vi "Periodic Tasks.vi"(8 "error in":errorcluster) -> ()   [LabVIEW 2014]
doc: "This VI runs in parallel to other tasks. It can contain as many user-defined periodic loops as you need. These can carry out PID or other sorts of timed response."
uses:
  <vilib>/Rock Robotics/WPI/Solenoid/WPI_SolenoidValue.ctl
  <vilib>/Rock Robotics/WPI/Joystick/WPI_JoystickGetSetRefNum.vi
  <vilib>/Rock Robotics/WPI/RobotDrive/WPI_RobotDriveGetSetRefNum.vi
  Global 1.vi
  <vilib>/Rock Robotics/WPI/Solenoid/WPI_SolenoidSetEnum.vi
  <vilib>/Rock Robotics/Network Tables/SD Write Numeric Array.vi
  <vilib>/Rock Robotics/Network Tables/SD Write Number.vi
  <vilib>/Rock Robotics/Network Tables/SD Read Boolean.vi
  <vilib>/addons/control/pid/pid.llb/PID (DBL).vi
  <vilib>/addons/control/pid/NI_PID_pid.lvlib
panel:
  out "Switch Pressed":bool
  out "Fudge":dbl
  out "Potentiometer Voltage":dbl
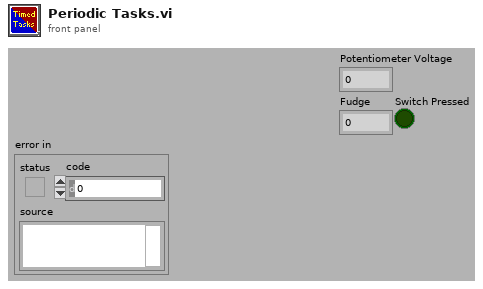
[diagram p1: front panel]
types:
  T1 = typedef "WPI_EncoderDevRef.ctl" = cluster{"DevStatus":errorcluster, "EncoderIndex":T2, "CounterIndex":T3, "DistancePerCount":dbl, "Decoding Type":T4}
  T2 = typedef "FPGA_EncoderIdx.ctl" = enum8{"Enc 0", "Enc 1", "Enc 2", "Enc 3", "Enc 4", "Enc 5", "Enc 6", "Enc 7", "Invalid"}
  T3 = typedef "FPGA_CounterCtrSystemIndex.ctl" = enum8{"Ctr 0", "Ctr 1", "Ctr 2", "Ctr 3", "Ctr 4", "Ctr 5", "Ctr 6", "Ctr 7", "Invalid"}
  T4 = typedef "WPI_EncoderType.ctl" = enum16{"1x", "2x", "4x"}
  T5 = typedef "WPI_JoystickDevRef.ctl" = cluster{"Device":T6}
  T6 = typedef "WPI_JoystickDeviceEnum.ctl" = enum16{"USB 0", "USB 1", "USB 2", "USB 3", "USB 4", "USB 5"}
  T7 = typedef "WPI_RobotDriveDevRef.ctl" = cluster{"DevStatus":errorcluster, "Motors[]":T8[], "Square Inputs":bool, "Max Output":dbl}
  T8 = typedef "WPI_MotorControlDeviceRef.ctl" = cluster{"DeviceStatus":errorcluster, "Type":T9, "PWM":cluster{"Controller":T10, "PWM Channel":T11, "DeadBand":T12}, "CAN":cluster{"Device Number":u8, "Control Mode":T13, "Semaphore":T14, "Max Vout":dbl, "TalonSRX Control Mode":T15}, "Invert":bool, "TransformRef":T16, "InvTransformRef":T16}
  T9 = typedef "WPI_MotorControlType.ctl" = enum16{"PWM", "CAN", "CANTalonSRX"}
  T10 = typedef "FPGA_TypedefDigitalModule.ctl" = enum16{"Controller 1"}
  T11 = typedef "FPGA_DIOPWMChannel.ctl" = enum8{"PWM 0", "PWM 1", "PWM 2", "PWM 3", "PWM 4", "PWM 5", "PWM 6", "PWM 7", "PWM 8", "PWM 9", "PWM MXP 0", "PWM MXP 1", "PWM MXP 2", "PWM MXP 3", "PWM MXP 4", "PWM MXP 5", "PWM MXP 6", "PWM MXP 7", "PWM MXP 8", "PWM MXP 9", "Invalid"}
  T12 = typedef "WPI_PWMDeadband.ctl" = cluster{"Name":string, "maxPositivePwm":i32, "minPositivePwm":i32, "centerPwm":i32, "maxNegativePwm":i32, "minNegativePwm":i32, "angularRange":u16}
  T13 = typedef "WPI_CANJaguar_ControlMode.ctl" = enum8{"Percent VBus", "Current", "Speed", "Position", "Voltage"}
  T14 = typedef "Semaphore RefNum" = refnum<k1>
  T15 = typedef "WPI_CANTalonSRX_APIControlMode.ctl" = enum8{"Percent VBus", "Speed", "Position", "Slave", "Unchanged / Invalid"}
  T16 = typedef "WPI_PWMTransform_ConPane.ctl" = refnum<vi>
  T17 = cluster{"JoystickDevRef":T5, "RobotDriveDevRef":T7}
  T18 = cluster{"proportional gain (Kc)":dbl, "integral time (Ti, min)":dbl, "derivative time (Td, min)":dbl}
  T19 = typedef "WPI_SolenoidValue.ctl" = enum16{"Off", "On", "Forward", "Reverse"}
  T20 = typedef "WPI_SolenoidDevRef.ctl" = cluster{"DevStatus":errorcluster, "Pneumatics Control Module":u8, "Forward Solenoid Channel":T21, "Reverse Solenoid Channel":T21}
  T21 = typedef "WPI_SolenoidChannel.ctl" = enum8{"Solenoid 0", "Solenoid 1", "Solenoid 2", "Solenoid 3", "Solenoid 4", "Solenoid 5", "Solenoid 6", "Solenoid 7", "Invalid"}
  T22 = typedef "WPI_SwitchDevRef.ctl" = cluster{"DevStatus":errorcluster, "DIO Channel":T23, "Controller":T10, "CntIndex":T3, "Normally Closed":bool}
  T23 = typedef "FPGA_DIOChannel.ctl" = enum8{"DIO 0", "DIO 1", "DIO 2", "DIO 3", "DIO 4", "DIO 5", "DIO 6", "DIO 7", "DIO 8", "DIO 9", "DIO MXP 0", "DIO MXP 1", "DIO MXP 2", "DIO MXP 3", "DIO MXP 4", "DIO MXP 5", "DIO MXP 6", "DIO MXP 7", "DIO MXP 8", "DIO MXP 9", "DIO MXP 10", "DIO MXP 11", "DIO MXP 12", "DIO MXP 13", "DIO MXP 14", "DIO MXP 15", "Invalid"}
  T24 = typedef "WPI_PotentiometerDevRef.ctl" = cluster{"DevStatus":errorcluster, "Controller":T25, "Analog Channel":T26, "Invert Output":bool}
  T25 = typedef "FPGA_TypedefAnalogModule.ctl" = enum16{"Controller 1"}
  T26 = typedef "FPGA_AIChannel.ctl" = enum8{"AI 0", "AI 1", "AI 2", "AI 3", "AI MXP 0", "AI MXP 1", "AI MXP 2", "AI MXP 3", "Invalid"}
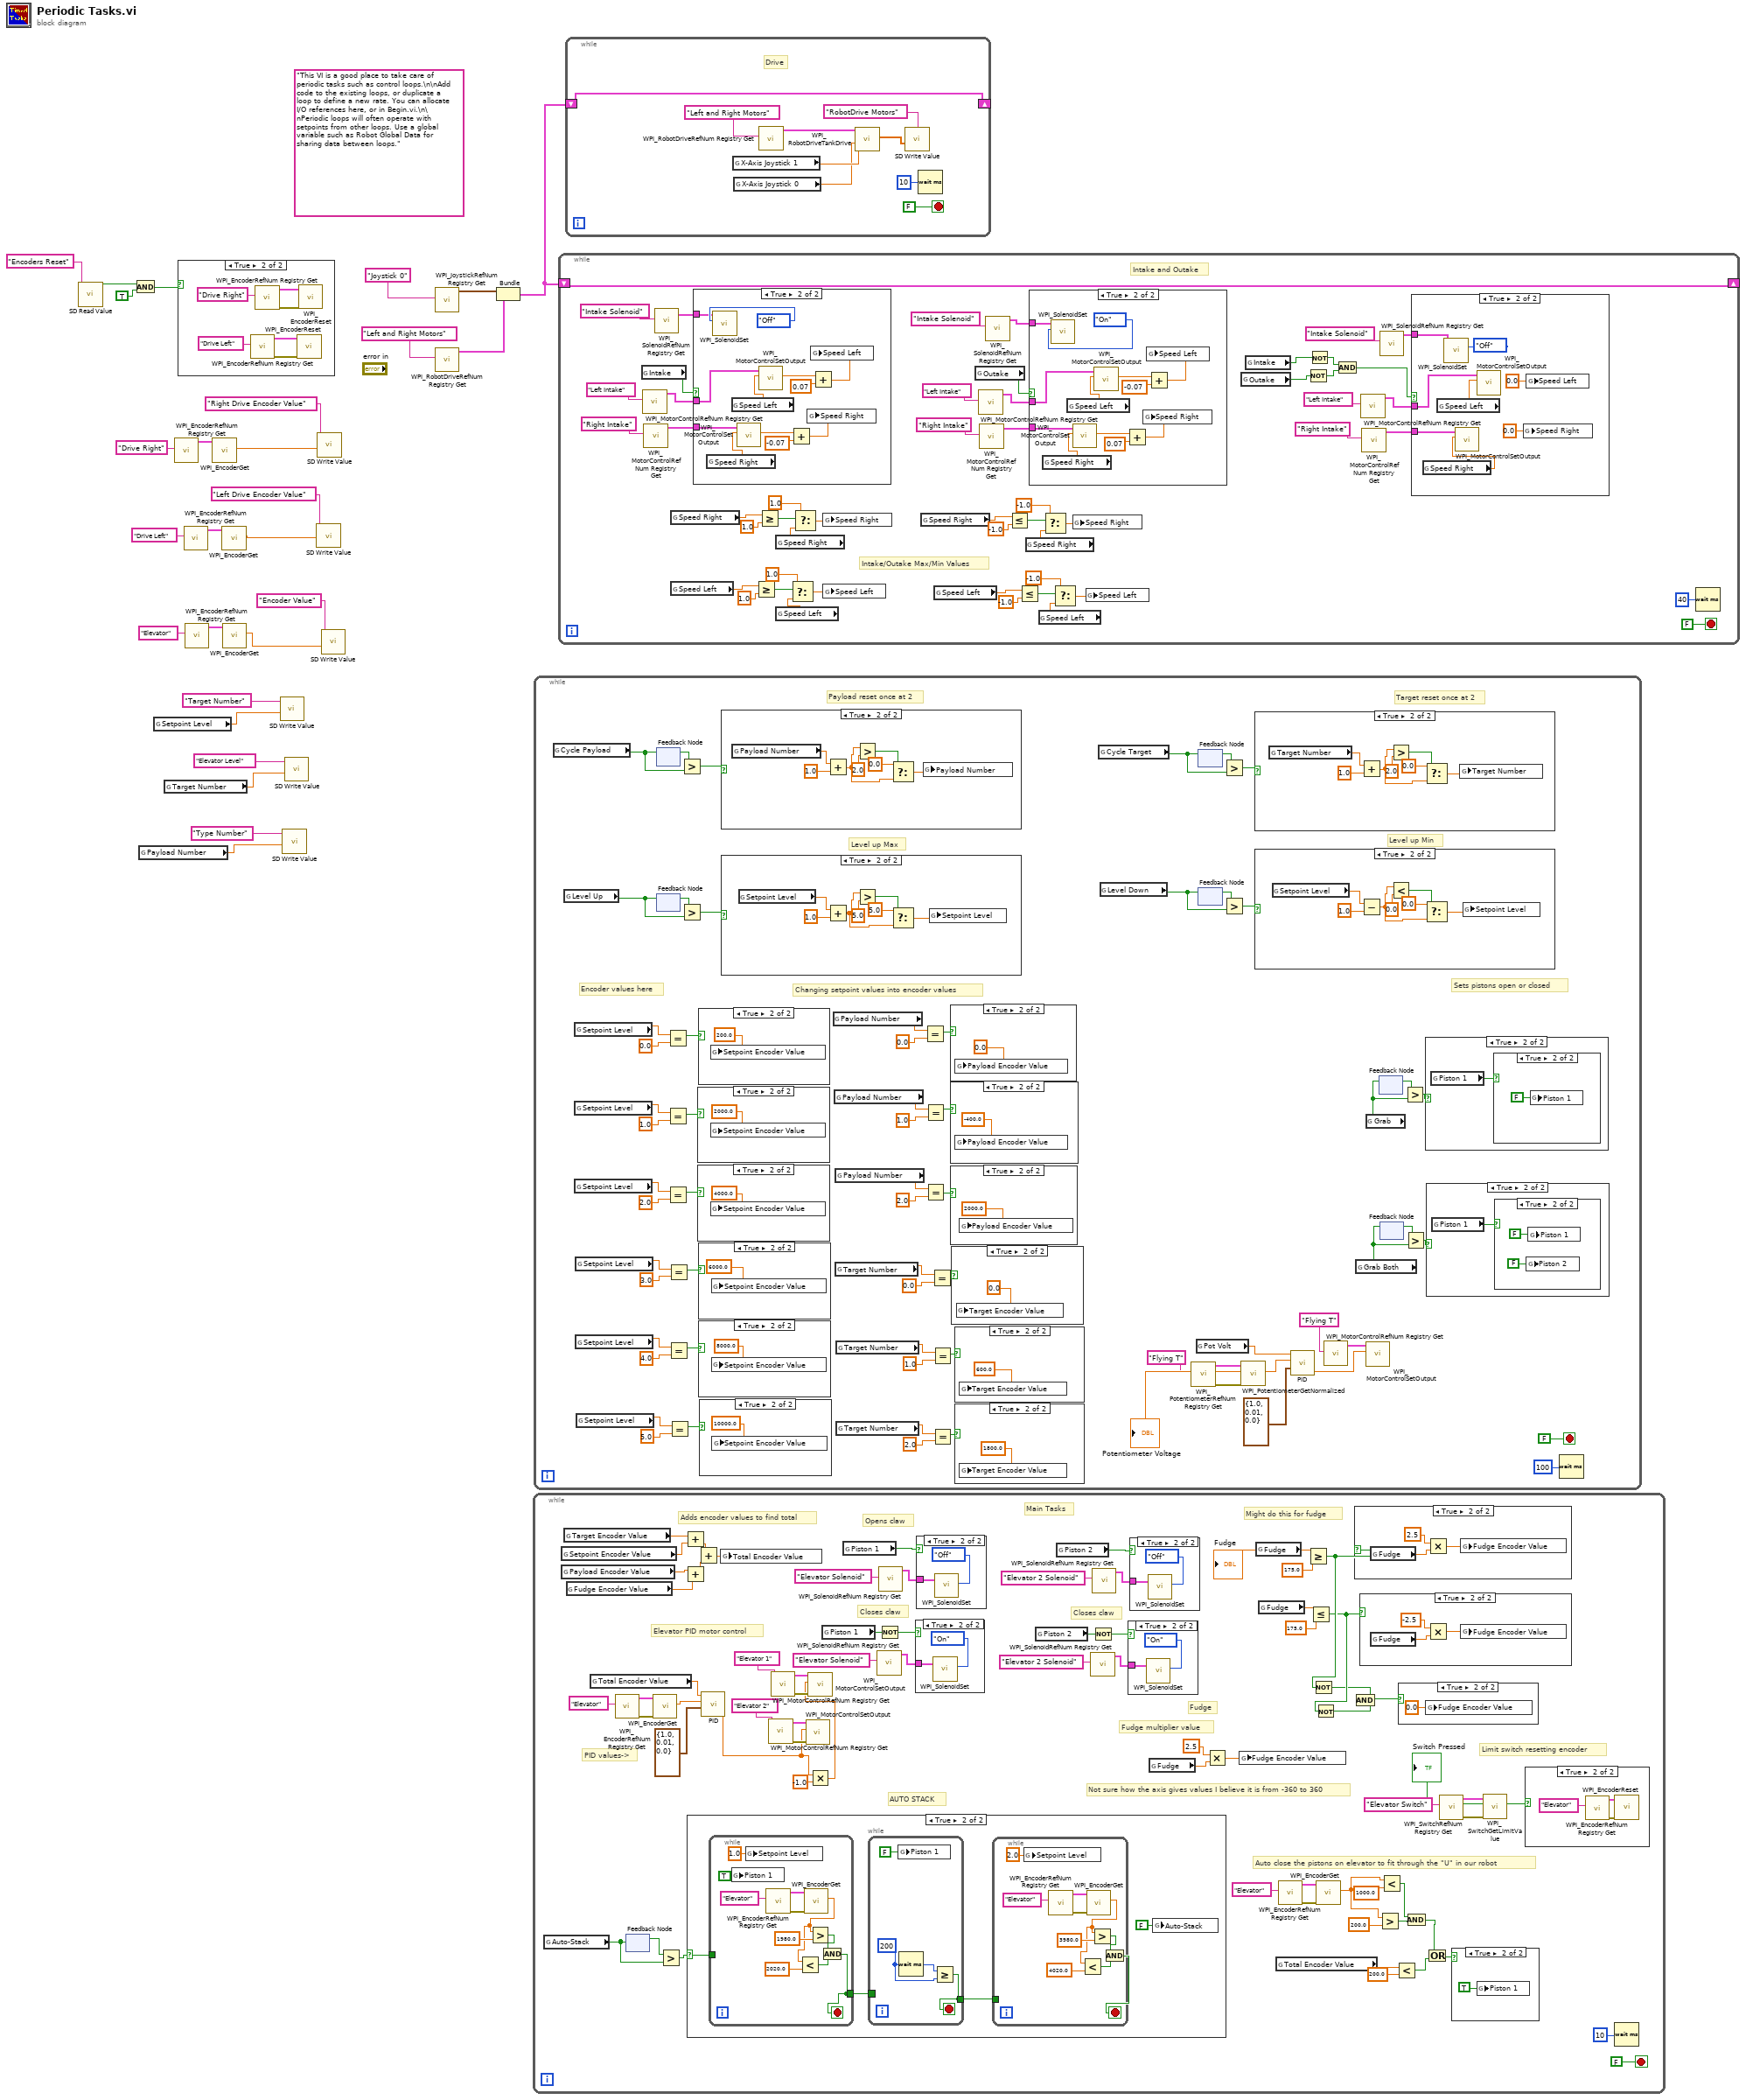
[diagram p0: block diagram]
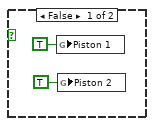
[diagram p14: hidden frame]
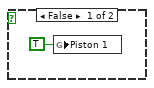
[diagram p16: hidden frame]
diagram:
  (unwired) "This VI is a good place to take care of periodic tasks such as control loops.\n\nAdd code to the existing loops, or duplicate a loop to define a new rate. You can allocate I/O references here, or in Begin.vi.\n\nPeriodic loops will often operate with setpoints from other loops. Use a global variable such as Robot Global Data for sharing data between loops."
  n1 = call-poly <vilib>:"SD Read Value.vi"("Name"="Encoders Reset") -> ("Boolean"=w2:bool)  [unwired: 8 in, 2 out]
  n2 = And(x=w2, y=TRUE) -> (x .and. y?=w1:bool)
  n3 = global read "Global 1.vi" "Payload Number"() -> (w7:dbl)
  n4 = global read "Global 1.vi" "Setpoint Level"() -> (w5:dbl)
  n5 = global read "Global 1.vi" "Target Number"() -> (w6:dbl)
  n6 = call <vilib>:"WPI_EncoderRefNum Registry Get.vi"("refnum name"="Drive Right") -> ("EncoderDevRef"=w19:T1)  [unwired: 9 in, 1 out]
  n7 = case shown="True" w1 {
    frame False {
    }
    frame True {
      n8 = call <vilib>:"WPI_EncoderRefNum Registry Get.vi"("refnum name"="Drive Left") -> ("error out"=w28:errorcluster, "EncoderDevRef"=w29:T1)  [unwired: 9 in]
      n9 = call <vilib>:"WPI_EncoderRefNum Registry Get.vi"("refnum name"="Drive Right") -> ("error out"=w31:errorcluster, "EncoderDevRef"=w30:T1)  [unwired: 9 in]
      n10 = call <vilib>:"WPI_EncoderReset.vi"("error in (no error)"=w28, "EncoderDevRef"=w29) -> ()  [unwired: 8 in, 2 out]
      n11 = call <vilib>:"WPI_EncoderReset.vi"("error in (no error)"=w31, "EncoderDevRef"=w30) -> ()  [unwired: 8 in, 2 out]
    }
  }
  n12 = call <vilib>:"WPI_EncoderRefNum Registry Get.vi"("refnum name"="Drive Left") -> ("EncoderDevRef"=w16:T1)  [unwired: 9 in, 1 out]
  n13 = call <vilib>:"WPI_EncoderRefNum Registry Get.vi"("refnum name"="Elevator") -> ("EncoderDevRef"=w14:T1)  [unwired: 9 in, 1 out]
  n14 = call <vilib>:"WPI_EncoderGet.vi"("EncoderDevRef"=w19) -> ("Distance"=w17:dbl)  [unwired: 5 in, 5 out]
  n15 = call <vilib>:"WPI_EncoderGet.vi"("EncoderDevRef"=w16) -> ("Distance"=w11:dbl)  [unwired: 5 in, 5 out]
  n16 = call <vilib>:"WPI_EncoderGet.vi"("EncoderDevRef"=w14) -> ("Distance"=w12:dbl)  [unwired: 5 in, 5 out]
  n17 = call-poly <vilib>:"SD Write Value.vi"("Numeric"=w5, "Name"="Target Number") -> ()  [unwired: 8 in, 2 out]
  n18 = call-poly <vilib>:"SD Write Value.vi"("Numeric"=w7, "Name"="Type Number") -> ()  [unwired: 8 in, 2 out]
  n19 = call-poly <vilib>:"SD Write Value.vi"("Numeric"=w6, "Name"="Elevator Level") -> ()  [unwired: 8 in, 2 out]
  n20 = call-poly <vilib>:"SD Write Value.vi"("Numeric"=w11, "Name"="Left Drive Encoder Value") -> ()  [unwired: 8 in, 2 out]
  n21 = call-poly <vilib>:"SD Write Value.vi"("Numeric"=w17, "Name"="Right Drive Encoder Value") -> ()  [unwired: 8 in, 2 out]
  n22 = call-poly <vilib>:"SD Write Value.vi"("Numeric"=w12, "Name"="Encoder Value") -> ()  [unwired: 8 in, 2 out]
  n23 = call <vilib>:"WPI_JoystickRefNum Registry Get.vi"("refnum name"="Joystick 0") -> ("JoystickDevRef"=w25:T5)  [unwired: 1 in, 9 out]
  n24 = call <vilib>:"WPI_RobotDriveRefNum Registry Get.vi"("refnum name"="Left and Right Motors") -> ("RobotDriveDevRef"=w24:T7)  [unwired: 1 in, 9 out]
  n25 = Bundle("JoystickDevRef"=w25, "RobotDriveDevRef"=w24) -> (w23:T17)  [unwired: 1 out]
  n26 = while {
    stop <- FALSE stop-if-true
    # "Auto close the pistons on elevator to fit through the \"U\" in our robot"
    # "Closes claw"
    # "Main Tasks"
    # "Limit switch resetting encoder"
    # "AUTO STACK"
    # "Might do this for fudge"
    # "Not sure how the axis gives values I believe it is from -360 to 360"
    # "Fudge multiplier value"
    # "Fudge"
    # "Elevator PID motor control"
    # "Adds encoder values to find total"
    # "Closes claw"
    # "Opens claw"
    # "PID values->"
    n27 = global read "Global 1.vi" "Auto-Stack"() -> (w61:bool)
    n28 = global read "Global 1.vi" "Setpoint Encoder Value"() -> (w100:dbl)
    n29 = global read "Global 1.vi" "Payload Encoder Value"() -> (w79:dbl)
    n30 = global read "Global 1.vi" "Target Encoder Value"() -> (w101:dbl)
    n31 = global read "Global 1.vi" "Fudge Encoder Value"() -> (w78:dbl)
    n32 = global read "Global 1.vi" "Total Encoder Value"() -> (w88:dbl)
    n33 = call <vilib>:"WPI_EncoderRefNum Registry Get.vi"("refnum name"="Elevator") -> ("error out"=w93:errorcluster, "EncoderDevRef"=w92:T1)  [unwired: 9 in]
    n34 = feedback-in #1(w61) -> ()
    n35 = feedback #1() -> (w62:bool)  [unwired: 1 in]
    n36 = call <vilib>:"WPI_EncoderGet.vi"("error in (no error)"=w93, "EncoderDevRef"=w92) -> ("Distance"=w89:dbl)  [unwired: 4 in, 5 out]
    n37 = Greater?(x=w62, y=w61) -> (0:w60:bool)
    n38 = Add(x=w101, y=w100) -> (x+y=w76:dbl)
    n39 = Add(x=w79, y=w78) -> (x+y=w77:dbl)
    n40 = case shown="True" w60 {
      selector: w60 -> [_ w115]
      frame False {
      }
      frame True {
        n41 = while {
          tunnel: w115 -> [_]
          tunnel: [w130] -> w114
          stop <- w130 stop-if-true
          n42 = global write "Global 1.vi" "Piston 1"(TRUE) -> ()
          n43 = global write "Global 1.vi" "Setpoint Level"(1.0 ("Setpoint Level")) -> ()
          n44 = call <vilib>:"WPI_EncoderRefNum Registry Get.vi"("refnum name"="Elevator") -> ("error out"=w138:errorcluster, "EncoderDevRef"=w137:T1)  [unwired: 9 in]
          n45 = call <vilib>:"WPI_EncoderGet.vi"("error in (no error)"=w138, "EncoderDevRef"=w137) -> ("Distance"=w134:dbl)  [unwired: 4 in, 5 out]
          n46 = Less?(x=w134, y=2020.0) -> (x < y?=w131:bool)
          n47 = Greater?(x=w134, y=1980.0) -> (0:w132:bool)
          n48 = And(x=w132, y=w131) -> (x .and. y?=w130:bool)
        }
        n49 = while {
          tunnel: w114 -> [_]
          tunnel: [w126] -> w113
          stop <- w126 stop-if-true
          w127 = u32 200 ("milliseconds to wait")
          n50 = global write "Global 1.vi" "Piston 1"(FALSE) -> ()
          n51 = Wait (ms)(milliseconds to wait=w127) -> (millisecond timer value=w128:u32)
          n52 = Greater Or Equal?(x=w128, y=w127) -> (x >= y?=w126:bool)
        }
        n53 = while {
          tunnel: w113 -> [_]
          stop <- w116 stop-if-true
          n54 = global write "Global 1.vi" "Setpoint Level"(2.0 ("Setpoint Level")) -> ()
          n55 = call <vilib>:"WPI_EncoderRefNum Registry Get.vi"("refnum name"="Elevator") -> ("error out"=w124:errorcluster, "EncoderDevRef"=w123:T1)  [unwired: 9 in]
          n56 = call <vilib>:"WPI_EncoderGet.vi"("error in (no error)"=w124, "EncoderDevRef"=w123) -> ("Distance"=w120:dbl)  [unwired: 4 in, 5 out]
          n57 = Less?(x=w120, y=4020.0) -> (x < y?=w117:bool)
          n58 = Greater?(x=w120, y=3980.0) -> (0:w118:bool)
          n59 = And(x=w118, y=w117) -> (x .and. y?=w116:bool)
        }
        n60 = global write "Global 1.vi" "Auto-Stack"(FALSE ("Auto-Stack")) -> ()
      }
    }
    n61 = Add(x=w76, y=w77) -> (x+y=w75:dbl)
    n62 = call-poly <vilib>:"PID.vi"("PID gains"=T18 {"proportional gain (Kc)"=1.0, "integral time (Ti, min)"=0.01, "derivative time (Td, min)"=0.0}, "process variable"=w89, "setpoint"=w88) -> ("output"=w86:dbl)  [unwired: 7 in, 1 out]
    n63 = global write "Global 1.vi" "Total Encoder Value"(w75) -> ()
    n64 = call <vilib>:"WPI_MotorControlRefNum Registry Get.vi"("refnum name"="Elevator 2") -> ("error out"=w94:errorcluster, "MotorControlDevRef"=w97:T8)  [unwired: 9 in]
    n65 = call <vilib>:"WPI_MotorControlRefNum Registry Get.vi"("refnum name"="Elevator 1") -> ("error out"=w95:errorcluster, "MotorControlDevRef"=w99:T8)  [unwired: 9 in]
    n66 = call <vilib>:"WPI_MotorControlSetOutput.vi"("error in (no error)"=w94, "Output"=w86, "MotorControlDevRef"=w97) -> ()  [unwired: 6 in, 3 out]
    n67 = Multiply(x=w86, y=-1.0) -> (x*y=w85:dbl)
    n68 = call <vilib>:"WPI_MotorControlSetOutput.vi"("error in (no error)"=w95, "Output"=w85, "MotorControlDevRef"=w99) -> ()  [unwired: 6 in, 3 out]
    n69 = global read "Global 1.vi" "Piston 1"() -> (w55:bool)
    n70 = global read "Global 1.vi" "Piston 1"() -> (w84:bool)
    n71 = call <vilib>:"WPI_SolenoidRefNum Registry Get.vi"("refnum name"="Elevator Solenoid") -> ("SolenoidDevRef"=w80:T20)  [unwired: 9 in, 1 out]
    n72 = Not(x=w55) -> (.not. x?=w54:bool)
    n73 = call <vilib>:"WPI_SolenoidRefNum Registry Get.vi"("refnum name"="Elevator Solenoid") -> ("SolenoidDevRef"=w82:T20)  [unwired: 9 in, 1 out]
    n74 = case shown="True" w54 {
      tunnel: w80 -> [_ w148]
      frame False {
      }
      frame True {
        n75 = call-poly <vilib>:"WPI_SolenoidSet.vi"("Value"=WPI_SolenoidValue."On", "SolenoidDevRef"=w148) -> ()  [unwired: 8 in, 2 out]
      }
    }
    n76 = case shown="True" w84 {
      tunnel: w82 -> [_ w150]
      frame False {
      }
      frame True {
        n77 = call-poly <vilib>:"WPI_SolenoidSet.vi"("Value"=WPI_SolenoidValue."Off", "SolenoidDevRef"=w150) -> ()  [unwired: 8 in, 2 out]
      }
    }
    n78 = global read "Global 1.vi" "Piston 2"() -> (w48:bool)
    n79 = global read "Global 1.vi" "Piston 2"() -> (w53:bool)
    n80 = call <vilib>:"WPI_SolenoidRefNum Registry Get.vi"("refnum name"="Elevator 2 Solenoid") -> ("SolenoidDevRef"=w49:T20)  [unwired: 9 in, 1 out]
    n81 = Not(x=w48) -> (.not. x?=w47:bool)
    n82 = call <vilib>:"WPI_SolenoidRefNum Registry Get.vi"("refnum name"="Elevator 2 Solenoid") -> ("SolenoidDevRef"=w51:T20)  [unwired: 9 in, 1 out]
    n83 = case shown="True" w47 {
      tunnel: w49 -> [_ w105]
      frame False {
      }
      frame True {
        n84 = call-poly <vilib>:"WPI_SolenoidSet.vi"("Value"=WPI_SolenoidValue."On", "SolenoidDevRef"=w105) -> ()  [unwired: 8 in, 2 out]
      }
    }
    n85 = case shown="True" w53 {
      tunnel: w51 -> [_ w107]
      frame False {
      }
      frame True {
        n86 = call-poly <vilib>:"WPI_SolenoidSet.vi"("Value"=WPI_SolenoidValue."Off", "SolenoidDevRef"=w107) -> ()  [unwired: 8 in, 2 out]
      }
    }
    n87 = global read "Global 1.vi" "Fudge"() -> (w72:dbl)
    n88 = Multiply(x=2.5, y=w72) -> (x*y=w74:dbl)
    n89 = global write "Global 1.vi" "Fudge Encoder Value"(w74) -> ()
    n90 = global read "Global 1.vi" "Fudge"() -> (w69:dbl)
    "Fudge" <- w69
    n91 = global read "Global 1.vi" "Fudge"() -> (w71:dbl)
    n92 = global read "Global 1.vi" "Total Encoder Value"() -> (w36:dbl)
    n93 = call <vilib>:"WPI_EncoderRefNum Registry Get.vi"("refnum name"="Elevator") -> ("error out"=w40:errorcluster, "EncoderDevRef"=w42:T1)  [unwired: 9 in]
    n94 = Greater Or Equal?(x=w69, y=175.0) -> (x >= y?=w67:bool)
    n95 = Less Or Equal?(x=w71, y=175.0) -> (x <= y?=w66:bool)
    n96 = Not(x=w67) -> (.not. x?=w65:bool)
    n97 = Not(x=w66) -> (.not. x?=w64:bool)
    n98 = call <vilib>:"WPI_EncoderGet.vi"("error in (no error)"=w40, "EncoderDevRef"=w42) -> ("Distance"=w38:dbl)  [unwired: 4 in, 5 out]
    n99 = And(x=w65, y=w64) -> (x .and. y?=w63:bool)
    n100 = case shown="True" w67 {
      frame False {
      }
      frame True {
        n101 = global read "Global 1.vi" "Fudge"() -> (w145:dbl)
        n102 = Multiply(x=2.5, y=w145) -> (x*y=w147:dbl)
        n103 = global write "Global 1.vi" "Fudge Encoder Value"(w147) -> ()
      }
    }
    n104 = case shown="True" w66 {
      frame False {
      }
      frame True {
        n105 = global read "Global 1.vi" "Fudge"() -> (w142:dbl)
        n106 = Multiply(x=-2.5, y=w142) -> (x*y=w144:dbl)
        n107 = global write "Global 1.vi" "Fudge Encoder Value"(w144) -> ()
      }
    }
    n108 = Greater?(x=w38, y=200.0) -> (0:w45:bool)
    n109 = Less?(x=w38, y=1000.0) -> (x < y?=w44:bool)
    n110 = Less?(x=w36, y=200.0) -> (x < y?=w34:bool)
    n111 = case shown="True" w63 {
      frame False {
      }
      frame True {
        n112 = global write "Global 1.vi" "Fudge Encoder Value"(0.0 ("Fudge Encoder Value")) -> ()
      }
    }
    n113 = And(x=w44, y=w45) -> (x .and. y?=w43:bool)
    n114 = Or(x=w43, y=w34) -> (x .or. y?=w46:bool)
    n115 = call <vilib>:"WPI_SwitchRefNum Registry Get.vi"("refnum name"="Elevator Switch") -> ("error out"=w58:errorcluster, "SwitchDevRef"=w57:T22)  [unwired: 9 in]
    n116 = case shown="True" w46 {
      frame False {
      }
      frame True {
        n117 = global write "Global 1.vi" "Piston 1"(TRUE ("Open")) -> ()
      }
    }
    n118 = call <vilib>:"WPI_SwitchGetLimitValue.vi"("error in (no error)"=w58, "SwitchDevRef"=w57) -> ("Switch Pressed"=w56:bool)  [unwired: 7 in, 2 out]
    "Switch Pressed" <- w56
    n119 = case shown="True" w56 {
      frame False {
      }
      frame True {
        n120 = call <vilib>:"WPI_EncoderRefNum Registry Get.vi"("refnum name"="Elevator") -> ("error out"=w110:errorcluster, "EncoderDevRef"=w109:T1)  [unwired: 9 in]
        n121 = call <vilib>:"WPI_EncoderReset.vi"("error in (no error)"=w110, "EncoderDevRef"=w109) -> ()  [unwired: 8 in, 2 out]
      }
    }
    n122 = Wait (ms)(milliseconds to wait=u32 10) -> ()  [unwired: 1 out]
  }
  n123 = while {
    stop <- FALSE stop-if-true
    # "Payload reset once at 2"
    # "Target reset once at 2"
    # "Level up Min"
    # "Level up Max"
    # "Sets pistons open or closed"
    # "Changing setpoint values into encoder values"
    # "Encoder values here"
    n124 = global read "Global 1.vi" "Cycle Payload"() -> (w214:bool)
    n125 = global read "Global 1.vi" "Level Up"() -> (w208:bool)
    n126 = global read "Global 1.vi" "Setpoint Level"() -> (w202:dbl)
    n127 = global read "Global 1.vi" "Setpoint Level"() -> (w198:dbl)
    n128 = global read "Global 1.vi" "Setpoint Level"() -> (w195:dbl)
    n129 = global read "Global 1.vi" "Setpoint Level"() -> (w192:dbl)
    n130 = global read "Global 1.vi" "Setpoint Level"() -> (w189:dbl)
    n131 = global read "Global 1.vi" "Setpoint Level"() -> (w186:dbl)
    n132 = feedback-in #2(w214) -> ()
    n133 = feedback #2() -> (w215:bool)  [unwired: 1 in]
    n134 = feedback #3() -> (w209:bool)  [unwired: 1 in]
    n135 = feedback-in #3(w208) -> ()
    n136 = Equal?(x=w202, y=0.0) -> (x = y?=w201:bool)
    n137 = Equal?(x=w198, y=1.0) -> (x = y?=w197:bool)
    n138 = Equal?(x=w195, y=2.0) -> (x = y?=w194:bool)
    n139 = Equal?(x=w192, y=3.0) -> (x = y?=w191:bool)
    n140 = Equal?(x=w189, y=4.0) -> (x = y?=w188:bool)
    n141 = Equal?(x=w186, y=5.0) -> (x = y?=w185:bool)
    n142 = Greater?(x=w215, y=w214) -> (0:w213:bool)
    n143 = Greater?(x=w209, y=w208) -> (0:w207:bool)
    n144 = case shown="True" w197 {
      frame False {
      }
      frame True {
        n145 = global write "Global 1.vi" "Setpoint Encoder Value"(2000.0 ("Setpoint Level")) -> ()
      }
    }
    n146 = case shown="True" w194 {
      frame False {
      }
      frame True {
        n147 = global write "Global 1.vi" "Setpoint Encoder Value"(4000.0 ("Setpoint Level")) -> ()
      }
    }
    n148 = case shown="True" w201 {
      frame False {
      }
      frame True {
        n149 = global write "Global 1.vi" "Setpoint Encoder Value"(200.0 ("Setpoint Level")) -> ()
      }
    }
    n150 = case shown="True" w191 {
      frame False {
      }
      frame True {
        n151 = global write "Global 1.vi" "Setpoint Encoder Value"(6000.0 ("Setpoint Level")) -> ()
      }
    }
    n152 = case shown="True" w188 {
      frame False {
      }
      frame True {
        n153 = global write "Global 1.vi" "Setpoint Encoder Value"(8000.0 ("Setpoint Level")) -> ()
      }
    }
    n154 = case shown="True" w185 {
      frame False {
      }
      frame True {
        n155 = global write "Global 1.vi" "Setpoint Encoder Value"(10000.0 ("Setpoint Level")) -> ()
      }
    }
    n156 = case shown="True" w213 {
      frame False {
      }
      frame True {
        n157 = global read "Global 1.vi" "Payload Number"() -> (w264:dbl)
        n158 = Add(x=w264, y=1.0) -> (x+y=w259:dbl)
        n159 = Greater?(x=w259, y=2.0) -> (0:w261:bool)
        n160 = Select(t=0.0, s=w261, f=w259) -> (s? t:f=w258:dbl)
        n161 = global write "Global 1.vi" "Payload Number"(w258) -> ()
      }
    }
    n162 = case shown="True" w207 {
      frame False {
      }
      frame True {
        n163 = global read "Global 1.vi" "Setpoint Level"() -> (w250:dbl)
        n164 = Add(x=w250, y=1.0) -> (x+y=w244:dbl)
        n165 = Greater?(x=w244, y=5.0) -> (0:w247:bool)
        n166 = Select(t=5.0, s=w247, f=w244) -> (s? t:f=w245:dbl)
        n167 = global write "Global 1.vi" "Setpoint Level"(w245) -> ()
      }
    }
    n168 = global read "Global 1.vi" "Payload Number"() -> (w183:dbl)
    n169 = global read "Global 1.vi" "Payload Number"() -> (w180:dbl)
    n170 = global read "Global 1.vi" "Payload Number"() -> (w177:dbl)
    n171 = global read "Global 1.vi" "Target Number"() -> (w174:dbl)
    n172 = global read "Global 1.vi" "Target Number"() -> (w171:dbl)
    n173 = global read "Global 1.vi" "Target Number"() -> (w168:dbl)
    n174 = Equal?(x=w183, y=0.0) -> (x = y?=w182:bool)
    n175 = Equal?(x=w180, y=1.0) -> (x = y?=w179:bool)
    n176 = Equal?(x=w177, y=2.0) -> (x = y?=w176:bool)
    n177 = Equal?(x=w174, y=0.0) -> (x = y?=w173:bool)
    n178 = Equal?(x=w171, y=1.0) -> (x = y?=w170:bool)
    n179 = Equal?(x=w168, y=2.0) -> (x = y?=w167:bool)
    n180 = case shown="True" w182 {
      frame False {
      }
      frame True {
        n181 = global write "Global 1.vi" "Payload Encoder Value"(0.0 ("Setpoint Level")) -> ()
      }
    }
    n182 = case shown="True" w179 {
      frame False {
      }
      frame True {
        n183 = global write "Global 1.vi" "Payload Encoder Value"(-400.0 ("Setpoint Level")) -> ()
      }
    }
    n184 = case shown="True" w176 {
      frame False {
      }
      frame True {
        n185 = global write "Global 1.vi" "Payload Encoder Value"(2000.0 ("Setpoint Level")) -> ()
      }
    }
    n186 = case shown="True" w173 {
      frame False {
      }
      frame True {
        n187 = global write "Global 1.vi" "Target Encoder Value"(0.0 ("Setpoint Level")) -> ()
      }
    }
    n188 = case shown="True" w170 {
      frame False {
      }
      frame True {
        n189 = global write "Global 1.vi" "Target Encoder Value"(600.0 ("Setpoint Level")) -> ()
      }
    }
    n190 = case shown="True" w167 {
      frame False {
      }
      frame True {
        n191 = global write "Global 1.vi" "Target Encoder Value"(1800.0 ("Setpoint Level")) -> ()
      }
    }
    n192 = global read "Global 1.vi" "Cycle Target"() -> (w211:bool)
    n193 = global read "Global 1.vi" "Level Down"() -> (w205:bool)
    n194 = call <vilib>:"WPI_PotentiometerRefNum Registry Get.vi"("refnum name"="Flying T") -> ("error out"=w160:errorcluster, "PotDevRef"=w162:T24)  [unwired: 9 in]
    n195 = global read "Global 1.vi" "Pot Volt"() -> (w152:dbl)
    n196 = feedback #4() -> (w212:bool)  [unwired: 1 in]
    n197 = feedback-in #4(w211) -> ()
    n198 = feedback #5() -> (w206:bool)  [unwired: 1 in]
    n199 = feedback-in #5(w205) -> ()
    n200 = Greater?(x=w212, y=w211) -> (0:w210:bool)
    n201 = Greater?(x=w206, y=w205) -> (0:w204:bool)
    n202 = call <vilib>:"WPI_PotentiometerGetNormalized.vi"("error in"=w160, "PotDevRef"=w162) -> ("Normalized Value"=w163:dbl)  [unwired: 7 in, 2 out]
    "Potentiometer Voltage" <- w163
    n203 = case shown="True" w210 {
      frame False {
      }
      frame True {
        n204 = global read "Global 1.vi" "Target Number"() -> (w257:dbl)
        n205 = Add(x=w257, y=1.0) -> (x+y=w252:dbl)
        n206 = Greater?(x=w252, y=2.0) -> (0:w254:bool)
        n207 = Select(t=0.0, s=w254, f=w252) -> (s? t:f=w251:dbl)
        n208 = global write "Global 1.vi" "Target Number"(w251) -> ()
      }
    }
    n209 = case shown="True" w204 {
      frame False {
      }
      frame True {
        n210 = global read "Global 1.vi" "Setpoint Level"() -> (w243:dbl)
        n211 = Subtract(x=w243, y=1.0) -> (x-y=w237:dbl)
        n212 = Less?(x=w237, y=0.0) -> (x < y?=w240:bool)
        n213 = Select(t=0.0, s=w240, f=w237) -> (s? t:f=w238:dbl)
        n214 = global write "Global 1.vi" "Setpoint Level"(w238) -> ()
      }
    }
    n215 = call-poly <vilib>:"PID.vi"("PID gains"=T18 {"proportional gain (Kc)"=1.0, "integral time (Ti, min)"=0.01, "derivative time (Td, min)"=0.0}, "process variable"=w163, "setpoint"=w152) -> ("dt out (s)"=w156:dbl)  [unwired: 7 in, 1 out]
    n216 = call <vilib>:"WPI_MotorControlRefNum Registry Get.vi"("refnum name"="Flying T") -> ("MotorControlDevRef"=w157:T8)  [unwired: 9 in, 1 out]
    n217 = global read "Global 1.vi" "Grab Both"() -> (w154:bool)
    n218 = global read "Global 1.vi" "Grab"() -> (w165:bool)
    n219 = call <vilib>:"WPI_MotorControlSetOutput.vi"("Output"=w156, "MotorControlDevRef"=w157) -> ()  [unwired: 7 in, 3 out]
    n220 = feedback #6() -> (w166:bool)  [unwired: 1 in]
    n221 = feedback-in #6(w165) -> ()
    n222 = feedback #7() -> (w155:bool)  [unwired: 1 in]
    n223 = feedback-in #7(w154) -> ()
    n224 = Greater?(x=w166, y=w165) -> (0:w164:bool)
    n225 = Greater?(x=w155, y=w154) -> (0:w153:bool)
    n226 = case shown="True" w164 {
      frame False {
      }
      frame True {
        n227 = global read "Global 1.vi" "Piston 1"() -> (w222:bool)
        n228 = case shown="True" w222 {
          frame False {
            n229 = global write "Global 1.vi" "Piston 1"(TRUE ("Piston 1")) -> ()
          }
          frame True {
            n230 = global write "Global 1.vi" "Piston 1"(FALSE ("Piston 1")) -> ()
          }
        }
      }
    }
    n231 = case shown="True" w153 {
      frame False {
      }
      frame True {
        n232 = global read "Global 1.vi" "Piston 1"() -> (w217:bool)
        n233 = case shown="True" w217 {
          frame False {
            n234 = global write "Global 1.vi" "Piston 1"(TRUE ("Piston 1")) -> ()
            n235 = global write "Global 1.vi" "Piston 2"(TRUE ("Piston 1")) -> ()
          }
          frame True {
            n236 = global write "Global 1.vi" "Piston 2"(FALSE ("Piston 1")) -> ()
            n237 = global write "Global 1.vi" "Piston 1"(FALSE ("Piston 1")) -> ()
          }
        }
      }
    }
    n238 = Wait (ms)(milliseconds to wait=u32 100) -> ()  [unwired: 1 out]
  }
  n239 = while {
    shift-right: [w316] -> _
    shift-left: w23 -> [w316]
    stop <- FALSE stop-if-true
    # "Intake and Outake"
    # "Intake/Outake Max/Min Values"
    n240 = global read "Global 1.vi" "Intake"() -> (w315:bool)
    n241 = call <vilib>:"WPI_MotorControlRefNum Registry Get.vi"("refnum name"="Left Intake") -> ("MotorControlDevRef"=w311:T8)  [unwired: 9 in, 1 out]
    n242 = call <vilib>:"WPI_MotorControlRefNum Registry Get.vi"("refnum name"="Right Intake") -> ("MotorControlDevRef"=w312:T8)  [unwired: 9 in, 1 out]
    n243 = call <vilib>:"WPI_SolenoidRefNum Registry Get.vi"("refnum name"="Intake Solenoid") -> ("SolenoidDevRef"=w265:T20)  [unwired: 9 in, 1 out]
    n244 = global read "Global 1.vi" "Speed Right"() -> (w294:dbl)
    n245 = global read "Global 1.vi" "Speed Left"() -> (w282:dbl)
    n246 = case shown="True" w315 {
      tunnel: w312 -> [_ w348]
      tunnel: w311 -> [_ w339]
      tunnel: w265 -> [_ w337]
      frame False {
      }
      frame True {
        n247 = global read "Global 1.vi" "Speed Right"() -> (w344:dbl)
        n248 = call-poly <vilib>:"WPI_SolenoidSet.vi"("Value"=WPI_SolenoidValue."Off", "SolenoidDevRef"=w337) -> ()  [unwired: 8 in, 2 out]
        n249 = global read "Global 1.vi" "Speed Left"() -> (w340:dbl)
        n250 = call <vilib>:"WPI_MotorControlSetOutput.vi"("Output"=w344, "MotorControlDevRef"=w348) -> ("Motor Output"=w347:dbl)  [unwired: 7 in, 2 out]
        n251 = call <vilib>:"WPI_MotorControlSetOutput.vi"("Output"=w340, "MotorControlDevRef"=w339) -> ("Motor Output"=w343:dbl)  [unwired: 7 in, 2 out]
        n252 = Add(x=w347, y=-0.07) -> (x+y=w345:dbl)
        n253 = global write "Global 1.vi" "Speed Right"(w345) -> ()
        n254 = Add(x=w343, y=0.07) -> (x+y=w341:dbl)
        n255 = global write "Global 1.vi" "Speed Left"(w341) -> ()
      }
    }
    n256 = Greater Or Equal?(x=w282, y=1.0) -> (x >= y?=w280:bool)
    n257 = Greater Or Equal?(x=w294, y=1.0) -> (x >= y?=w292:bool)
    n258 = global read "Global 1.vi" "Speed Right"() -> (w290:dbl)
    n259 = global read "Global 1.vi" "Speed Left"() -> (w278:dbl)
    n260 = Select(t=1.0, s=w280, f=w278) -> (s? t:f=w279:dbl)
    n261 = Select(t=1.0, s=w292, f=w290) -> (s? t:f=w291:dbl)
    n262 = global write "Global 1.vi" "Speed Right"(w291) -> ()
    n263 = global write "Global 1.vi" "Speed Left"(w279) -> ()
    n264 = global read "Global 1.vi" "Speed Right"() -> (w288:dbl)
    n265 = global read "Global 1.vi" "Speed Left"() -> (w276:dbl)
    n266 = global read "Global 1.vi" "Outake"() -> (w310:bool)
    n267 = call <vilib>:"WPI_MotorControlRefNum Registry Get.vi"("refnum name"="Left Intake") -> ("MotorControlDevRef"=w306:T8)  [unwired: 9 in, 1 out]
    n268 = call <vilib>:"WPI_MotorControlRefNum Registry Get.vi"("refnum name"="Right Intake") -> ("MotorControlDevRef"=w307:T8)  [unwired: 9 in, 1 out]
    n269 = call <vilib>:"WPI_SolenoidRefNum Registry Get.vi"("refnum name"="Intake Solenoid") -> ("SolenoidDevRef"=w267:T20)  [unwired: 9 in, 1 out]
    n270 = Less Or Equal?(x=w288, y=-1.0) -> (x <= y?=w286:bool)
    n271 = Less Or Equal?(x=w276, y=-1.0) -> (x <= y?=w274:bool)
    n272 = global read "Global 1.vi" "Speed Right"() -> (w284:dbl)
    n273 = case shown="True" w310 {
      tunnel: w307 -> [_ w336]
      tunnel: w306 -> [_ w327]
      tunnel: w267 -> [_ w326]
      frame False {
      }
      frame True {
        n274 = global read "Global 1.vi" "Speed Right"() -> (w332:dbl)
        n275 = call-poly <vilib>:"WPI_SolenoidSet.vi"("Value"=WPI_SolenoidValue."On", "SolenoidDevRef"=w326) -> ()  [unwired: 8 in, 2 out]
        n276 = global read "Global 1.vi" "Speed Left"() -> (w328:dbl)
        n277 = call <vilib>:"WPI_MotorControlSetOutput.vi"("Output"=w332, "MotorControlDevRef"=w336) -> ("Motor Output"=w335:dbl)  [unwired: 7 in, 2 out]
        n278 = call <vilib>:"WPI_MotorControlSetOutput.vi"("Output"=w328, "MotorControlDevRef"=w327) -> ("Motor Output"=w331:dbl)  [unwired: 7 in, 2 out]
        n279 = Add(x=w335, y=0.07) -> (x+y=w333:dbl)
        n280 = global write "Global 1.vi" "Speed Right"(w333) -> ()
        n281 = Add(x=w331, y=-0.07) -> (x+y=w329:dbl)
        n282 = global write "Global 1.vi" "Speed Left"(w329) -> ()
      }
    }
    n283 = global read "Global 1.vi" "Speed Left"() -> (w272:dbl)
    n284 = Select(t=-1.0, s=w286, f=w284) -> (s? t:f=w285:dbl)
    n285 = Select(t=-1.0, s=w274, f=w272) -> (s? t:f=w273:dbl)
    n286 = global write "Global 1.vi" "Speed Right"(w285) -> ()
    n287 = global write "Global 1.vi" "Speed Left"(w273) -> ()
    n288 = global read "Global 1.vi" "Outake"() -> (w298:bool)
    n289 = global read "Global 1.vi" "Intake"() -> (w299:bool)
    n290 = Not(x=w298) -> (.not. x?=w296:bool)
    n291 = Not(x=w299) -> (.not. x?=w297:bool)
    n292 = And(x=w297, y=w296) -> (x .and. y?=w295:bool)
    n293 = call <vilib>:"WPI_MotorControlRefNum Registry Get.vi"("refnum name"="Left Intake") -> ("MotorControlDevRef"=w302:T8)  [unwired: 9 in, 1 out]
    n294 = call <vilib>:"WPI_MotorControlRefNum Registry Get.vi"("refnum name"="Right Intake") -> ("MotorControlDevRef"=w303:T8)  [unwired: 9 in, 1 out]
    n295 = call <vilib>:"WPI_SolenoidRefNum Registry Get.vi"("refnum name"="Intake Solenoid") -> ("SolenoidDevRef"=w301:T20)  [unwired: 9 in, 1 out]
    n296 = case shown="True" w295 {
      tunnel: w303 -> [_ w324]
      tunnel: w302 -> [_ w323]
      tunnel: w301 -> [_ w322]
      frame False {
      }
      frame True {
        n297 = global read "Global 1.vi" "Speed Right"() -> (w319:dbl)
        n298 = global read "Global 1.vi" "Speed Left"() -> (w320:dbl)
        n299 = call-poly <vilib>:"WPI_SolenoidSet.vi"("Value"=WPI_SolenoidValue."Off", "SolenoidDevRef"=w322) -> ()  [unwired: 8 in, 2 out]
        n300 = call <vilib>:"WPI_MotorControlSetOutput.vi"("Output"=w319, "MotorControlDevRef"=w324) -> ()  [unwired: 7 in, 3 out]
        n301 = call <vilib>:"WPI_MotorControlSetOutput.vi"("Output"=w320, "MotorControlDevRef"=w323) -> ()  [unwired: 7 in, 3 out]
        n302 = global write "Global 1.vi" "Speed Right"(0.0 ("Speed Right")) -> ()
        n303 = global write "Global 1.vi" "Speed Left"(0.0 ("Speed Left")) -> ()
      }
    }
    n304 = Wait (ms)(milliseconds to wait=u32 40) -> ()  [unwired: 1 out]
  }
  n305 = while {
    shift-right: [w355] -> _
    shift-left: w23 -> [w355]
    stop <- FALSE stop-if-true
    # "Drive"
    n306 = global read "Global 1.vi" "X-Axis Joystick 1"() -> (w350:dbl)
    n307 = global read "Global 1.vi" "X-Axis Joystick 0"() -> (w349:dbl)
    n308 = call <vilib>:"WPI_RobotDriveRefNum Registry Get.vi"("refnum name"="Left and Right Motors") -> ("RobotDriveDevRef"=w353:T7)  [unwired: 1 in, 9 out]
    n309 = call <vilib>:"WPI_RobotDriveTankDrive.vi"("Right axis value"=w349, "Left axis value"=w350, "RobotDriveDevRef"=w353) -> ("Motor Values"=w351:dbl[])  [unwired: 6 in, 2 out]
    n310 = call-poly <vilib>:"SD Write Value.vi"("Numeric Array"=w351, "Name"="RobotDrive Motors") -> ()  [unwired: 8 in, 2 out]
    n311 = Wait (ms)(milliseconds to wait=u32 10) -> ()  [unwired: 1 out]
  }
